vi "Length_1.vi"() -> ()   [LabVIEW 2020]
uses:
  Support/Controls/Cmd_Mouse Popup.ctl
  Support/Controls/Clst_Initialize Input.ctl
  Support/Controls/Clst_Result inspec.ctl
  Support/Controls/Cmd_Var Data IO.ctl
  Variables/Global_Cal Info.vi
panel:
  in  "Measured_ADJ":string[][](table) caption="조정후"
  out "최소범위":string
  out "STD set":string[][](table) caption="○ 기준기 조합 (값)"
  in  "Measured 2":string[][](table) caption="틈새교정"
  in  "표시방식":string(combo)
  out "단위":string
  out "최대범위":string
  in  "Spec 변경":bool
  in  "Random":bool
  out "Resolution":string[][](table) caption="Spec"
  out "Spec":string[][](table)
  out "제목":string
  out "에러 출력":errorcluster
  out "Condition":string[][](table) caption="2. 직선성 시험"
  in  "최소눈금":string(combo)
  in  "Measured":string[][](table) caption="조정전"
  out "Load?":bool
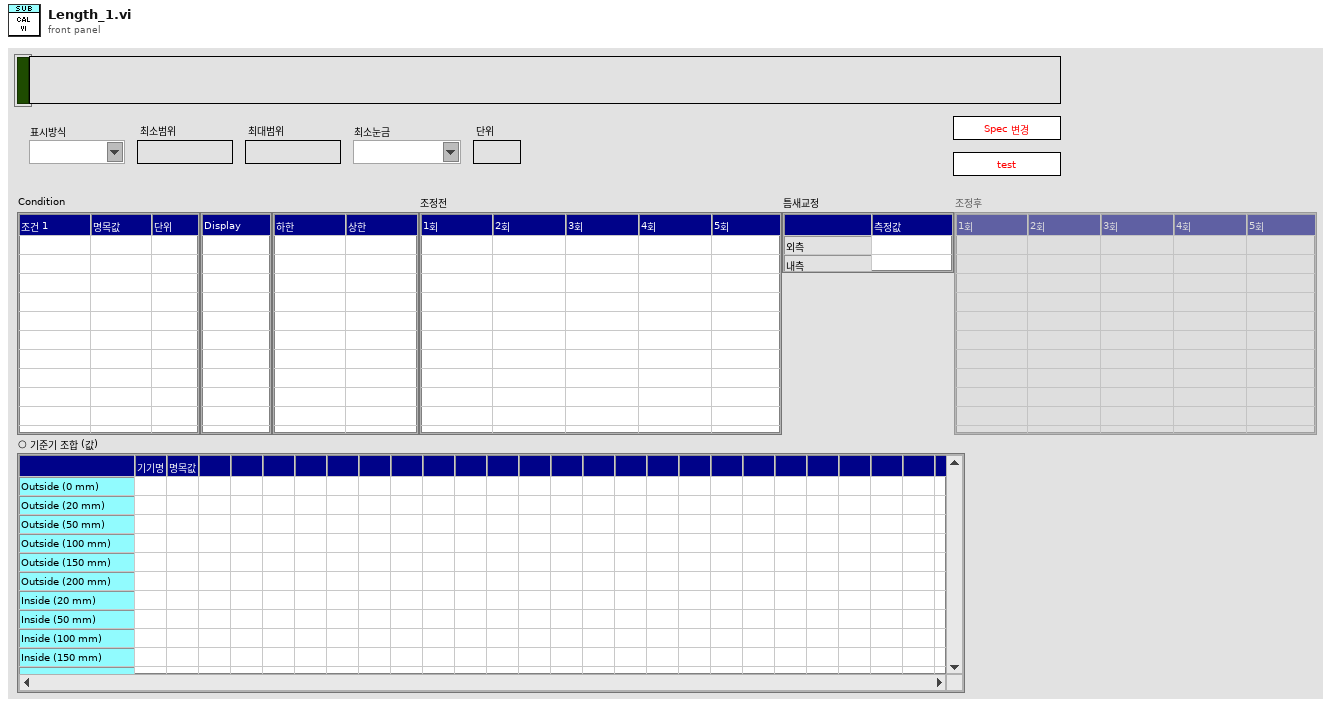
[diagram p1: front panel]
types:
  T1 = typedef "Cmd_Mouse Popup.ctl" = enum16{"활성화", "메뉴선택"}
  T2 = cluster{"Shift":bool, "Ctrl":bool, "Alt":bool, "Cmd":bool, "Opt":bool}
  T3 = typedef "Clst_Initialize Input.ctl" = cluster{"Initialize 1":cluster{"Condition":refnum<vi>[], "Spec":refnum<vi>[], "Measured":refnum<vi>[], "Resolution":refnum<vi>[], "Func_ext":string, "제목":refnum<vi>, "Measured_ADJ":refnum<vi>[]}, "Initialize 2":cluster{"문자열":refnum<vi>[], "콤보박스":refnum<vi>[], "링":refnum<vi>[], "열거형":refnum<vi>[], "테이블":refnum<vi>[], "여러열":refnum<vi>[], "디지털(DBL)":refnum<vi>[], "3D string":refnum<vi>[], "ctrl":refnum<vi>[], "boolean":refnum<vi>[]}}
  T4 = typedef "Clst_Result inspec.ctl" = cluster{"분해능":string, "문자열 1":string, "문자열 2":string, "숫자형 1":i32, "숫자형 2":i32, "숫자형 3":dbl, "문자배열 1D":string[], "문자배열 2D":string[][], "문자배열 3D":string[][][], "문자배열 4D":string[][][][], "불리언 1D":bool[]}
  T5 = typedef "Cmd_Var Data IO.ctl" = enum16{"Condition", "Condition Default", "Condition_Temp", "Resolution", "Resolution Default", "Resolution Old", "Spec", "Spec Default", "Spec Old", "Spec Temp", "Result", "Result2", "Result3", "Result_Temp", "Result_ADJ", "Result_ADJ2", "STD1", "STD2", "STD3", "STD4", "STD5", "STD Temp", "CMC", "CMC Default"}
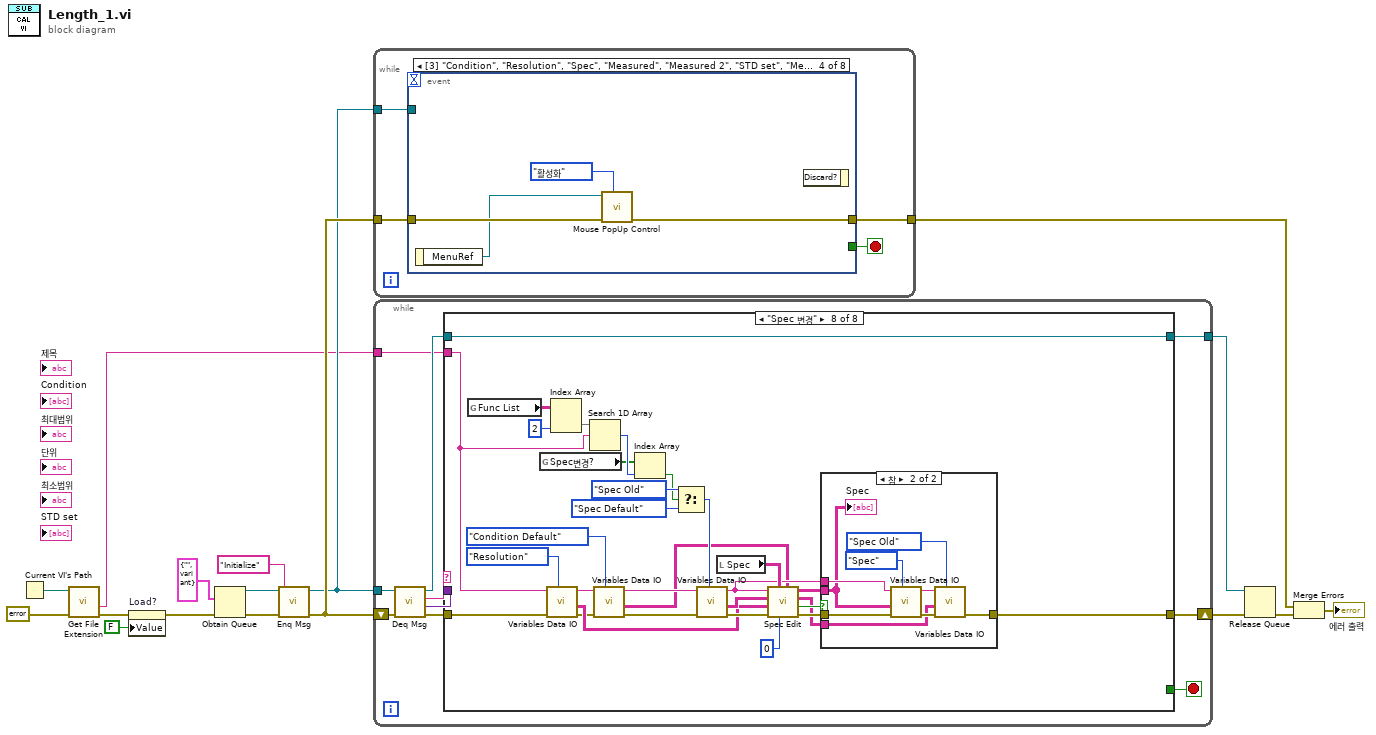
[diagram p0: block diagram]
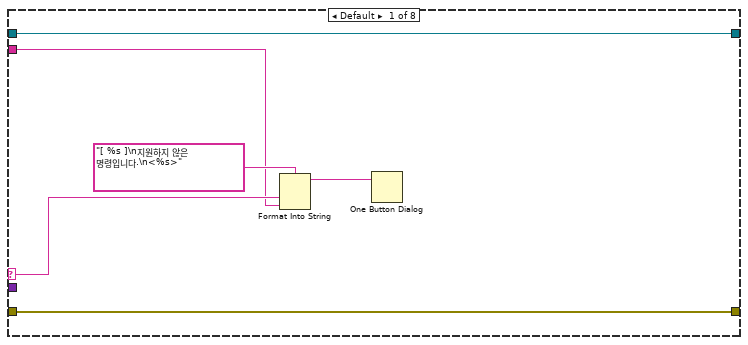
[diagram p2: hidden frame]
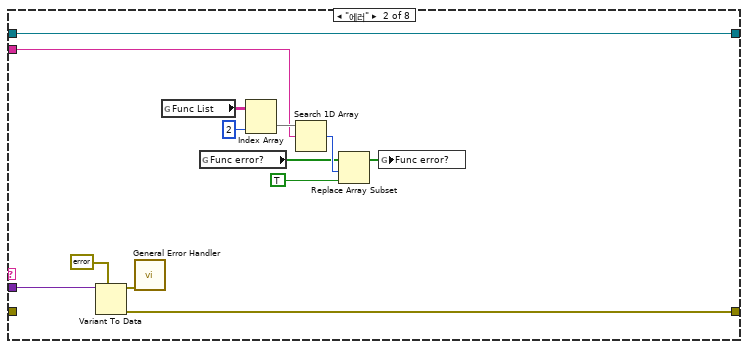
[diagram p3: hidden frame]
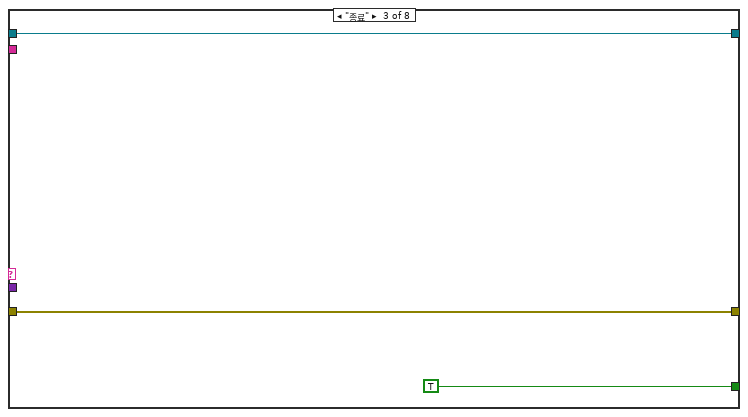
[diagram p4: hidden frame]
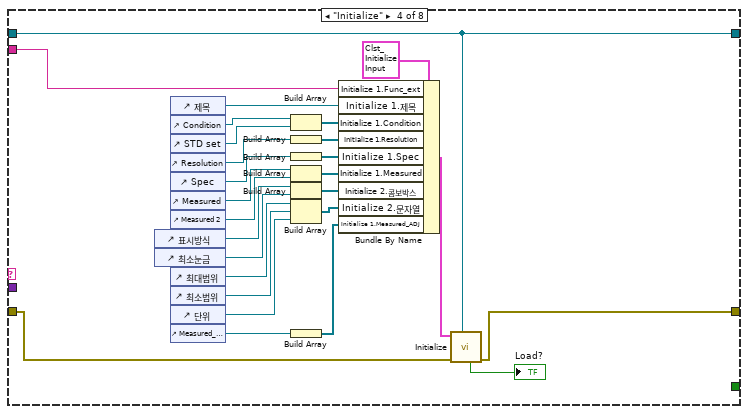
[diagram p5: hidden frame]
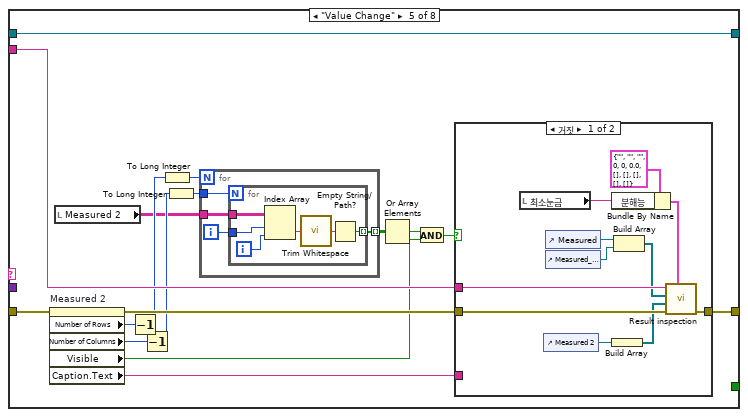
[diagram p6: hidden frame]
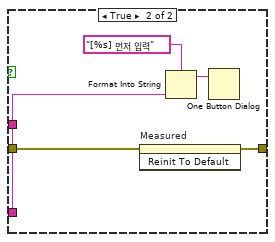
[diagram p7: hidden frame]
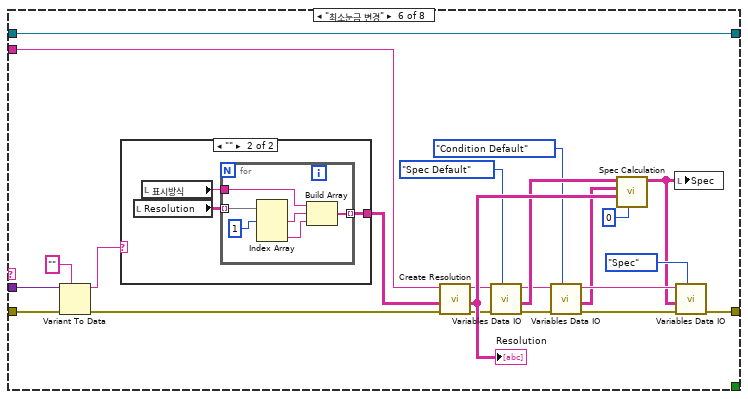
[diagram p8: hidden frame]
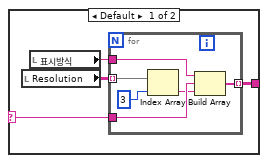
[diagram p9: hidden frame]
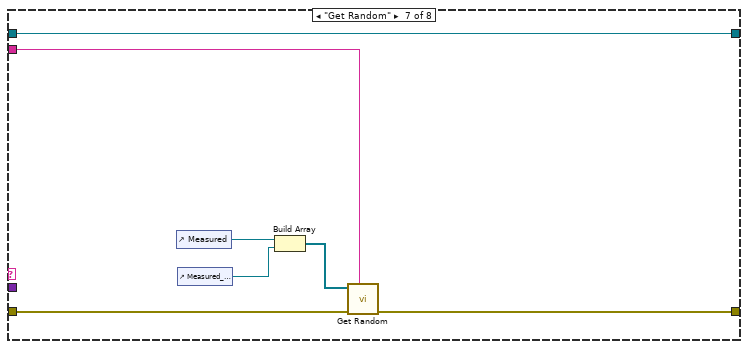
[diagram p10: hidden frame]
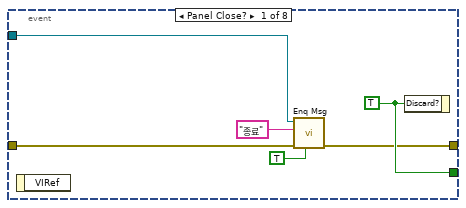
[diagram p12: hidden frame]
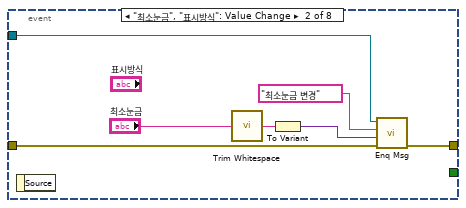
[diagram p13: hidden frame]
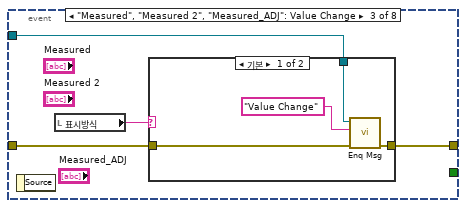
[diagram p14: hidden frame]
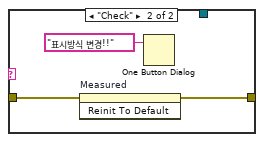
[diagram p15: hidden frame]
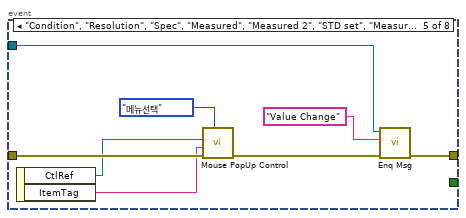
[diagram p16: hidden frame]
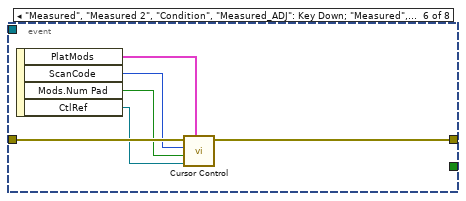
[diagram p17: hidden frame]
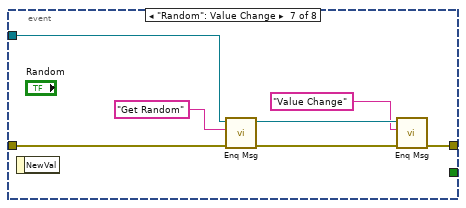
[diagram p18: hidden frame]
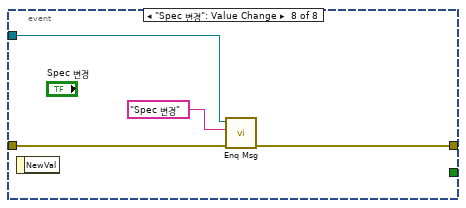
[diagram p19: hidden frame]
diagram:
  n1 = Current VI's Path() -> (path=w5:path)
  n2 = call <vilib>:"Get File Extension.vi"("error in (no error)"=errorcluster {"status"=FALSE, "code"=0, "source"=""} ("에러 상수"), "file"=w5) -> ("error out"=w3:errorcluster, "filename without extension"=w4:string)  [unwired: 5 in, 3 out]
  n3 = property on="Load?" class="Bool (엄격한)"(error in=w3, "Value"=FALSE ("Load?")) -> (error out=w2:errorcluster)  [unwired: 1 in, 1 out]
  n4 = Obtain Queue(element data type=cluster{"메세지":string, "값":variant} {"메세지"="", "값"=variant} ("Message Cluster"), error in (no error)=w2) -> (queue out=w14:refnum<queue>, error out=w16:errorcluster)  [unwired: 3 in, 1 out]
  n5 = call "Enq Msg.vi"("에러 입력(에러 없음)"=w16, "메세지"="Initialize", "큐 입력"=w14) -> ("에러 출력"=w15:errorcluster, "큐 출력"=w12:refnum<queue>)  [unwired: 7 in]
  n6 = while {
    tunnel: w15 -> [w19]
    tunnel: w12 -> [w20]
    tunnel: [w18] -> w9
    stop <- w21 stop-if-true
    n7 = event shown="[3] \"Condition\", \"Resolution\", \"Spec\", \"Measured\", \"Measured 2\", \"STD set\", \"Measured_ADJ\": 바로 가기 메뉴 활성화?" {
      selector: _ -> [_ _ _ _ _ _ _ _]
      dyn-events: _ -> [_ _ _ _ _ _ _ _]
      timeout: _ -> [_ _ _ _ _ _ _ _]
      tunnel: [w27 _ _ _ _ _ _ _] -> w21
      tunnel: w20 -> [w25 w33 w38 _ w50 _ w68 w72]
      tunnel: w19 -> [w26 w34 w36 w49 w57 w63 w69 w73]
      tunnel: [w23 w32 w37 w48 w51 w62 w64 w71] -> w18
      event Panel Close? {
        w27 = TRUE ("버림?")
        n8 = event-data() -> ()  [unwired: 1 in, 1 out]
        n9 = call "Enq Msg.vi"("우선순위 메시지?"=TRUE, "에러 입력(에러 없음)"=w26, "메세지"="종료", "큐 입력"=w25) -> ("에러 출력"=w23:errorcluster)  [unwired: 6 in, 1 out]
        n10 = event-data("Discard?"=w27) -> ()  [unwired: 1 in, 1 out]
      }
      event "최소눈금", "표시방식": Value Change {
        n11 = event-data() -> ()  [unwired: 1 in, 1 out]
        n12 = call <vilib>:"Trim Whitespace.vi"("string"="최소눈금") -> ("trimmed string"=w30:string)  [unwired: 1 in]
        n13 = To Variant(anything=w30) -> (Variant=w28:variant)
        n14 = call "Enq Msg.vi"("에러 입력(에러 없음)"=w34, "값"=w28, "메세지"="최소눈금 변경", "큐 입력"=w33) -> ("에러 출력"=w32:errorcluster)  [unwired: 6 in, 1 out]
      }
      event "Measured", "Measured 2", "Measured_ADJ": Value Change {
        n15 = event-data() -> ()  [unwired: 1 in, 1 out]
        n16 = local read "표시방식"() -> (w35:string)
        n17 = case shown="기본" w35 {
          tunnel: w38 -> [w42 _]
          tunnel: [w41 w43] -> w37
          tunnel: w36 -> [w40 w44]
          frame Default {
            n18 = call "Enq Msg.vi"("에러 입력(에러 없음)"=w40, "메세지"="Value Change", "큐 입력"=w42) -> ("에러 출력"=w41:errorcluster)  [unwired: 7 in, 1 out]
          }
          frame "Check" {
            n19 = invoke on="Measured" class="Tbl (엄격한)" method="Reinit To Default"(error in=w44) -> (error out=w43:errorcluster)  [unwired: 2 in, 2 out]
            n20 = One Button Dialog(message="표시방식 변경!!" ("메시지")) -> ()  [unwired: 1 in, 1 out]
          }
        }
      }
      event "Condition", "Resolution", "Spec", "Measured", "Measured 2", "STD set", "Measured_ADJ": Shortcut Menu Activation? {
        n21 = event-data() -> ("MenuRef"=w47:refnum<k9>)  [unwired: 1 in]
        n22 = call "Mouse PopUp Control.vi"("type"=Cmd_Mouse_Popup."활성화", "error in"=w49, "메뉴 참조"=w47) -> ("error out"=w48:errorcluster)  [unwired: 8 in]
        n23 = event-data() -> ()  [unwired: 2 in, 1 out]
      }
      event "Condition", "Resolution", "Spec", "Measured", "Measured 2", "STD set", "Measured_ADJ": Shortcut Menu Selection (User) {
        n24 = event-data() -> ("CtlRef"=w55:refnum<vi>, "ItemTag"=w54:string)  [unwired: 1 in]
        n25 = call "Mouse PopUp Control.vi"("type"=Cmd_Mouse_Popup."메뉴선택", "error in"=w57, "아이템 태그"=w54, "Tbl 참조 번호"=w55) -> ("error out"=w52:errorcluster)  [unwired: 7 in]
        n26 = call "Enq Msg.vi"("에러 입력(에러 없음)"=w52, "메세지"="Value Change", "큐 입력"=w50) -> ("에러 출력"=w51:errorcluster)  [unwired: 7 in, 1 out]
      }
      event "Measured", "Measured 2", "Condition", "Measured_ADJ": Key Down; "Measured", "Measured 2", "Condition", "Measured_ADJ": Key Repeat {
        n27 = event-data() -> ("PlatMods"=w58:T2, "ScanCode"=w61:i16, "Mods.Num Pad"=w60:bool, "CtlRef"=w59:refnum<vi>)  [unwired: 1 in]
        n28 = call "Cursor Control.vi"("플랫폼 조합키"=w58, "참조"=w59, "Num Pad"=w60, "ScanCode"=w61, "error in"=w63) -> ("error out"=w62:errorcluster)  [unwired: 5 in, 1 out]
      }
      event "Random": Value Change {
        n29 = event-data() -> ()  [unwired: 1 in, 1 out]
        n30 = call "Enq Msg.vi"("에러 입력(에러 없음)"=w69, "메세지"="Get Random", "큐 입력"=w68) -> ("에러 출력"=w67:errorcluster, "큐 출력"=w66:refnum<queue>)  [unwired: 7 in]
        n31 = call "Enq Msg.vi"("에러 입력(에러 없음)"=w67, "메세지"="Value Change", "큐 입력"=w66) -> ("에러 출력"=w64:errorcluster)  [unwired: 7 in, 1 out]
      }
      event "Spec 변경": Value Change {
        n32 = event-data() -> ()  [unwired: 1 in, 1 out]
        n33 = call "Enq Msg.vi"("에러 입력(에러 없음)"=w73, "메세지"="Spec 변경", "큐 입력"=w72) -> ("에러 출력"=w71:errorcluster)  [unwired: 7 in, 1 out]
      }
    }
  }
  n34 = while {
    shift-right: [w84] -> w11
    shift-left: w15 -> [w83]
    tunnel: w12 -> [w81]
    tunnel: [w76] -> w10
    tunnel: w4 -> [w75]
    stop <- w77 stop-if-true
    n35 = call "Deq Msg.vi"("에러 입력(에러 없음)"=w83, "큐 입력"=w81) -> ("에러 출력"=w82:errorcluster, "값"=w78:variant, "메세지"=w80:string, "큐 출력"=w79:refnum<queue>)  [unwired: 6 in]
    n36 = case shown="\"Spec 변경\"" w80 {
      selector: w80 -> [w86 _ _ _ _ _ _ _]
      tunnel: w82 -> [w90 _ w106 w112 w146 w198 w221 w248]
      tunnel: [w90 w100 w106 w110 w149 w191 w222 w251] -> w84
      tunnel: w79 -> [w89 w99 w104 w119 w150 w199 w225 w255]
      tunnel: w78 -> [_ w101 _ _ _ w197 _ _]
      tunnel: [_ _ TRUE ("버림?") _ _ _ _ _] -> w77
      tunnel: [w89 w99 w104 w119 w150 w199 w225 w255] -> w76
      tunnel: w75 -> [w85 w91 _ w120 w148 w195 w220 w233]
      frame Default {
        n37 = Format Into String(format string="[ %s ]\n지원하지 않은 명령입니다.\n<%s>" ("메시지"), w86, w85) -> (resulting string=w87:string)  [unwired: 2 in, 1 out]
        n38 = One Button Dialog(message=w87) -> ()  [unwired: 1 in, 1 out]
      }
      frame "에러" {
        n39 = Variant To Data(type=errorcluster {"status"=FALSE, "code"=0, "source"=""} ("에러 출력"), Variant=w101) -> (data=w103:errorcluster, error out=w100:errorcluster)  [unwired: 1 in]
        n40 = call <vilib>:"General Error Handler.vi"("error in (no error)"=w103) -> ()  [unwired: 10 in, 5 out]
        n41 = global read "Global_Cal Info.vi" "Func List"() -> (w93:string[][])
        n42 = global read "Global_Cal Info.vi" "Func error?"() -> (w96:bool[])
        n43 = Index Array(array=w93, index (col)=2 ("비활성화된 인덱스 (열)")) -> (element=w94:string[])  [unwired: 1 in]
        n44 = Search 1D Array(1D array=w94, element=w91) -> (index of element=w97:i32)  [unwired: 1 in]
        n45 = Replace Array Subset(array=w96, new element=TRUE ("새 원소/부분배열"), index=w97) -> (w98:bool[])
        n46 = global write "Global_Cal Info.vi" "Func error?"(w98) -> ()
      }
      frame "종료" {
      }
      frame "Initialize" {
        n47 = control-ref of="표시방식"() -> (w118:refnum<vi>)
        n48 = control-ref of="최소눈금"() -> (w127:refnum<vi>)
        n49 = control-ref of="제목"() -> (w125:refnum<vi>)
        n50 = control-ref of="Condition"() -> (w131:refnum<vi>)
        n51 = control-ref of="STD set"() -> (w113:refnum<vi>)
        n52 = control-ref of="Resolution"() -> (w121:refnum<vi>)
        n53 = control-ref of="Spec"() -> (w124:refnum<vi>)
        n54 = control-ref of="Measured"() -> (w128:refnum<vi>)
        n55 = control-ref of="Measured 2"() -> (w114:refnum<vi>)
        n56 = control-ref of="최대범위"() -> (w111:refnum<vi>)
        n57 = control-ref of="최소범위"() -> (w115:refnum<vi>)
        n58 = control-ref of="단위"() -> (w117:refnum<vi>)
        n59 = control-ref of="Measured_ADJ"() -> (w109:refnum<vi>)
        n60 = Build Array(w131, w113) -> (w130:refnum<vi>[])
        n61 = Build Array(w121) -> (w122:refnum<vi>[])
        n62 = Build Array(w124) -> (w123:refnum<vi>[])
        n63 = Build Array(w128, w114) -> (w129:refnum<vi>[])
        n64 = Build Array(w118, w127) -> (w126:refnum<vi>[])
        n65 = Build Array(w111, w115, w117) -> (w116:refnum<vi>[])
        n66 = Build Array(w109) -> (w108:refnum<vi>[])
        n67 = Bundle By Name(cluster=T3 {"Initialize 1"={"Condition"=[], "Spec"=[], "Measured"=[], "Resolution"=[], "Func_ext"="", "제목"=refnum, "Measured_ADJ"=[]}, "Initialize 2"={"문자열"=[], "콤보박스"=[], "링"=[], "열거형"=[], "테이블"=[], "여러열"=[], "디지털(DBL)"=[], "3D string"=[], "ctrl"=[], "boolean"=[]}} ("입력 클러스터"), "Initialize 1.Func_ext"=w120, "Initialize 1.제목"=w125, "Initialize 1.Condition"=w130, "Initialize 1.Resolution"=w122, "Initialize 1.Spec"=w123, "Initialize 1.Measured"=w129, "Initialize 2.콤보박스"=w126, "Initialize 2.문자열"=w116, "Initialize 1.Measured_ADJ"=w108) -> (w132:T3)
        n68 = call "Initialize.vi"("큐 입력"=w119, "error in"=w112, "입력 클러스터"=w132) -> ("error out"=w110:errorcluster, "Load?"=→"Load?":bool)  [unwired: 5 in, 2 out]
      }
      frame "Value Change" {
        n69 = property on="Measured 2" class="Tbl (엄격한)"(error in=w146) -> (error out=w145:errorcluster, "Number of Rows"=w147:u32, "Number of Columns"=w142:u32, "Visible"=w136:bool, "Caption.Text"=w144:string)  [unwired: 1 in, 1 out]
        n70 = local read "Measured 2"() -> (w134:string[][])
        n71 = Decrement(x=w147) -> (x-1=w143:u32)
        n72 = Decrement(x=w142) -> (x-1=w141:u32)
        n73 = To Long Integer(number=w143) -> (32bit integer=w139:i32)
        n74 = To Long Integer(number=w141) -> (32bit integer=w140:i32)
        n75 = for {
          N: w139 -> [_]
          tunnel: w134 -> [w153]
          tunnel: w140 -> [w154]
          tunnel: [w152] -> w138 mode=indexing
          i -> [w151]
          n76 = for {
            N: w154 -> [_]
            tunnel: w153 -> [w158]
            tunnel: [w159] -> w152 mode=indexing
            tunnel: w151 -> [w156]
            i -> [w155]
            n77 = Index Array(array=w158, index (row)=w156, index (col)=w155) -> (element=w157:string)
            n78 = call <vilib>:"Trim Whitespace.vi"("string"=w157) -> ("trimmed string"=w160:string)  [unwired: 1 in]
            n79 = Empty String/Path?(string/path=w160) -> (empty?=w159:bool)
          }
        }
        n80 = Or Array Elements(Boolean array=w138) -> (logical OR=w137:bool)
        n81 = And(x=w137, y=w136) -> (x .and. y?=w135:bool)
        n82 = case shown="거짓" w135 {
          tunnel: [w171 w172] -> w149
          tunnel: w148 -> [w170 _]
          tunnel: w145 -> [w164 w173]
          tunnel: w144 -> [_ w176]
          frame False {
            n83 = local read "최소눈금"() -> (w166:string)
            n84 = control-ref of="Measured 2"() -> (w163:refnum<vi>)
            n85 = control-ref of="Measured"() -> (w169:refnum<vi>)
            n86 = control-ref of="Measured_ADJ"() -> (w161:refnum<vi>)
            n87 = Bundle By Name(cluster=T4 {"분해능"="", "문자열 1"="", "문자열 2"="", "숫자형 1"=0, "숫자형 2"=0, "숫자형 3"=0.0, "문자배열 1D"=[], "문자배열 2D"=[], "문자배열 3D"=[], "문자배열 4D"=[], "불리언 1D"=[]} ("입력 클러스터"), "분해능"=w166) -> (w165:T4)
            n88 = Build Array(w163) -> (w162:refnum<vi>[])
            n89 = Build Array(w169, w161) -> (w168:refnum<vi>[])
            n90 = call "Result inspection.vi"("입력 클러스터"=w165, "error in"=w164, "Ref. Data (excluded)"=w162, "Ref. Data (Inspection)"=w168, "Func ext"=w170) -> ("error out"=w171:errorcluster)  [unwired: 3 in, 3 out]
          }
          frame True {
            n91 = invoke on="Measured" class="Tbl (엄격한)" method="Reinit To Default"(error in=w173) -> (error out=w172:errorcluster)  [unwired: 2 in, 2 out]
            n92 = Format Into String(format string="[%s] 먼저 입력" ("포맷 문자열"), w176) -> (resulting string=w174:string)  [unwired: 2 in, 1 out]
            n93 = One Button Dialog(message=w174) -> ()  [unwired: 1 in, 1 out]
          }
        }
      }
      frame "최소눈금 변경" {
        n94 = Variant To Data(error in=w198, type="", Variant=w197) -> (data=w184:string, error out=w186:errorcluster)
        n95 = case shown="\"\"" w184 {
          selector: w184 -> [w200 _]
          tunnel: [w203 w212] -> w185
          frame Default {
            n96 = local read "Resolution"() -> (w202:string[][])
            n97 = local read "표시방식"() -> (w201:string)
            n98 = for {
              tunnel: w202 -> [w209] mode=indexing
              tunnel: w200 -> [w208]
              tunnel: [w206] -> w203 mode=indexing
              tunnel: w201 -> [w205]
              n99 = Index Array(array=w209, index=3 ("인덱스")) -> (element=w207:string)
              n100 = Build Array(w205, w208, w207) -> (w206:string[])
            }
          }
          frame "" {
            n101 = local read "Resolution"() -> (w211:string[][])
            n102 = local read "표시방식"() -> (w210:string)
            n103 = for {
              tunnel: w211 -> [w218] mode=indexing
              tunnel: [w217] -> w212 mode=indexing
              tunnel: w210 -> [w216]
              n104 = Index Array(array=w218, index #1=1 ("인덱스")) -> (element #1=w214:string, element #3=w213:string)  [unwired: 2 in, 1 out]
              n105 = Build Array(w216, w214, w213) -> (w217:string[])
            }
          }
        }
        n106 = call "Create Resolution.vi"("에러 입력(에러 없음)"=w186, "Resolution"=w185, "Func_ext"=w195) -> ("에러 출력"=w189:errorcluster, "Resolution Out"=w192:string[][], "Func_ext 출력"=w188:string)  [unwired: 6 in]
        "Resolution" <- w192
        n107 = call "Variables Data IO.vi"("Select"=Cmd_Var_Data_IO."Spec Default", "error in"=w189, "Func_ext"=w188) -> ("error out"=w181:errorcluster, "Data Out"=w187:string[][], "Func_ext Out"=w183:string)  [unwired: 6 in]
        n108 = call "Variables Data IO.vi"("Select"=Cmd_Var_Data_IO."Condition Default", "error in"=w181, "Func_ext"=w183) -> ("error out"=w180:errorcluster, "Data Out"=w178:string[][], "Func_ext Out"=w182:string)  [unwired: 6 in]
        n109 = call "Spec Calculation.vi"("기준값 열번호"=0 ("열번호(기준값)"), "Resolution"=w192, "Condition in"=w178, "Spec Default"=w187) -> ("Spec out"=w177:string[][])  [unwired: 6 in, 1 out]
        n110 = local write "Spec"(w177) -> ()
        n111 = call "Variables Data IO.vi"("Select"=Cmd_Var_Data_IO."Spec", "error in"=w180, "Data In"=w177, "Func_ext"=w182) -> ("error out"=w191:errorcluster)  [unwired: 5 in, 2 out]
      }
      frame "Get Random" {
        n112 = control-ref of="Measured"() -> (w224:refnum<vi>)
        n113 = control-ref of="Measured_ADJ"() -> (w219:refnum<vi>)
        n114 = Build Array(w224, w219) -> (w223:refnum<vi>[])
        n115 = call "Get Random.vi"("Func_Ext"=w220, "에러 입력"=w221, "Meas"=w223) -> ("에러 출력"=w222:errorcluster)  [unwired: 7 in, 1 out]
      }
      frame "Spec 변경" {
        n116 = global read "Global_Cal Info.vi" "Func List"() -> (w238:string[][])
        n117 = global read "Global_Cal Info.vi" "Spec변경?"() -> (w234:bool[])
        n118 = call "Variables Data IO.vi"("Select"=Cmd_Var_Data_IO."Resolution", "error in"=w248, "Func_ext"=w233) -> ("error out"=w231:errorcluster, "Data Out"=w242:string[][], "Func_ext Out"=w229:string)  [unwired: 6 in]
        n119 = Index Array(array=w238, index (col)=2 ("비활성화된 인덱스 (열)")) -> (element=w236:string[])  [unwired: 1 in]
        n120 = Search 1D Array(1D array=w236, element=w233) -> (index of element=w235:i32)  [unwired: 1 in]
        n121 = call "Variables Data IO.vi"("Select"=Cmd_Var_Data_IO."Condition Default", "error in"=w231, "Func_ext"=w229) -> ("error out"=w230:errorcluster, "Data Out"=w226:string[][], "Func_ext Out"=w228:string)  [unwired: 6 in]
        n122 = Index Array(array=w234, index=w235) -> (element=w239:bool)
        n123 = Select(t=Cmd_Var_Data_IO."Spec Old" ("Select"), s=w239, f=Cmd_Var_Data_IO."Spec Default" ("Select")) -> (s? t:f=w232:T5)
        n124 = call "Variables Data IO.vi"("Select"=w232, "error in"=w230, "Func_ext"=w228) -> ("error out"=w250:errorcluster, "Data Out"=w243:string[][], "Func_ext Out"=w244:string)  [unwired: 6 in]
        n125 = local read "Spec"() -> (w245:string[][])
        n126 = call "Spec Edit.vi"("Condition"=w226, "열번호(기준값)"=0, "Spec Value"=w245, "에러 입력(에러 없음)"=w250, "Resolution"=w242, "Spec Default"=w243, "Func_ext"=w244) -> ("에러 출력"=w252:errorcluster, "변경?"=w253:bool, "Spec Default out"=w247:string[][], "Spec 출력"=w254:string[][])  [unwired: 1 in]
        n127 = case shown="참" w253 {
          tunnel: w254 -> [_ w262]
          tunnel: w252 -> [w256 w265]
          tunnel: [w256 w260] -> w251
          tunnel: w244 -> [_ w263]
          tunnel: w247 -> [_ w258]
          frame False {
          }
          frame True {
            n128 = call "Variables Data IO.vi"("Select"=Cmd_Var_Data_IO."Spec", "error in"=w265, "Data In"=w262, "Func_ext"=w263) -> ("error out"=w261:errorcluster, "Func_ext Out"=w259:string)  [unwired: 5 in, 1 out]
            n129 = call "Variables Data IO.vi"("Select"=Cmd_Var_Data_IO."Spec Old", "error in"=w261, "Data In"=w258, "Func_ext"=w259) -> ("error out"=w260:errorcluster)  [unwired: 5 in, 2 out]
            "Spec" <- w262
          }
        }
      }
    }
  }
  n130 = Release Queue(queue=w10, error in (no error)=w11) -> (error out=w8:errorcluster)  [unwired: 1 in, 2 out]
  n131 = Merge Errors(w9, w8) -> (→"에러 출력":errorcluster)
